vi "write KPRO file.vi"(9 "Corrected Array in":dbl[][](array[numeric]), 10 "Generate Array Calc IK":bool, 11 "Path in":refnum<vi>) -> (1 "paths ok":bool, 3 "appended path":path)   [LabVIEW 2016]
uses:
  C/Program Files (x86)/National Instruments/LabVIEW 2016/user.lib/_OpenG.lib/file/file.llb/Strip Path - Traditional__ogtk.vi
  C/Program Files (x86)/National Instruments/LabVIEW 2016/user.lib/_OpenG.lib/file/file.llb/Build Path - Traditional__ogtk.vi
  <vilib>/Utility/file.llb/Write Delimited Spreadsheet (DBL).vi
panel:
  out "type":i16
  out "Value":path
  out "error out":errorcluster
  in  "error in (no error)":errorcluster
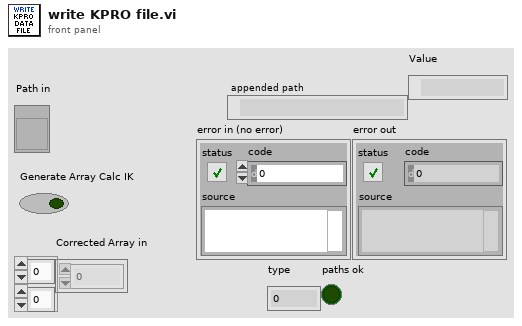
[diagram p1: front panel]
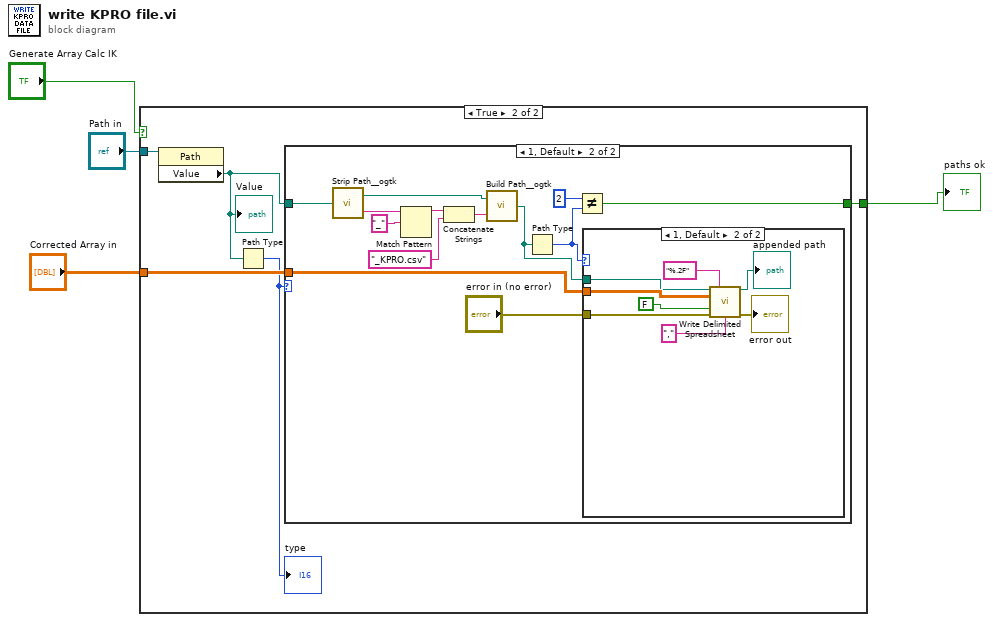
[diagram p0: block diagram]
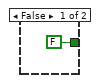
[diagram p2: hidden frame]
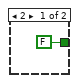
[diagram p3: hidden frame]
diagram:
  n1 = case shown="True" "Generate Array Calc IK" {
    tunnel: "Corrected Array in" -> [_ w10]
    tunnel: "Path in" -> [_ w9]
    tunnel: [FALSE w6] -> w1
    frame False {
    }
    frame True {
      n2 = property class="Path"(reference=w9) -> ("Value"=w8:path)  [unwired: 1 in, 2 out]
      "Value" <- w8
      n3 = Path Type(1:w8) -> (0:w7:i16)
      "type" <- w7
      n4 = case shown="1, Default" w7 {
        tunnel: w10 -> [_ w24]
        tunnel: w8 -> [_ w16]
        tunnel: [FALSE w12] -> w6
        frame 2 {
        }
        frame 1, Default {
          n5 = call-poly "Strip Path__ogtk.vi"("path"=w16) -> ("stripped path"=w23:path, "name"=w22:string)
          n6 = Match Pattern(string=w22, regular expression="_") -> (before substring=w20:string)  [unwired: 1 in, 3 out]
          n7 = Concatenate Strings(w20, "_KPRO.csv") -> (w19:string)
          n8 = call-poly "Build Path__ogtk.vi"("name or relative path"=w19, "base path"=w23) -> ("appended path"=w15:path)
          n9 = Path Type(1:w15) -> (0:w14:i16)
          n10 = Not Equal?(x=i16 2, y=w14) -> (x != y?=w12:bool)
          n11 = case shown="1, Default" w14 {
            tunnel: w24 -> [_ w32]
            tunnel: "error in (no error)" -> [_ w28]
            tunnel: w15 -> [_ w26]
            frame 2 {
            }
            frame 1, Default {
              n12 = call-poly <vilib>:"Write Delimited Spreadsheet.vi"("file path (dialog if empty)"=w26, "format (%.3f)"="%.2F", "2D data"=w32, "append to file? (new file:F)"=FALSE, "error in (no error)"=w28, "delimiter (\\t)"="," ("delimiter (\\t)")) -> ("new file path (Not A Path if cancelled)"=→"appended path":path, "error out"=→"error out":errorcluster)  [unwired: 8 in]
            }
          }
        }
      }
    }
  }
  "paths ok" <- w1
